vi "wsConnection_cycle_index.vi"() -> ()   [LabVIEW 2013]
uses:
  <vilib>/MediaMongrels Ltd/WebSockets/WebSockets/WebSockets.lvlib
panel:
  out "Numeric":i32
  in  "Frequency":dbl min=0.0
  in  "stop":bool
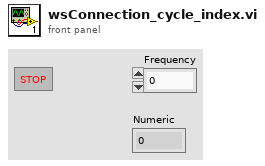
[diagram p1: front panel]
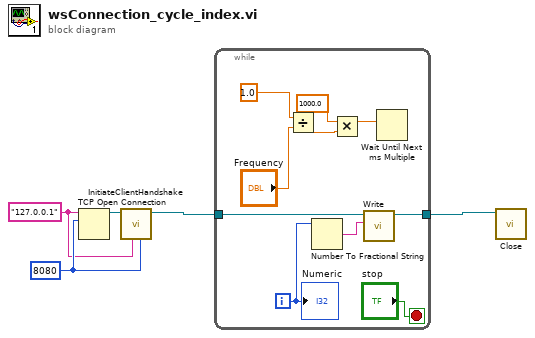
[diagram p0: block diagram]
diagram:
  w4 = "127.0.0.1"
  w5 = 8080
  n1 = TCP Open Connection(address=w4, remote port or service name=w5) -> (connection ID=w3:refnum<k5>)  [unwired: 3 in, 1 out]
  n2 = call <vilib>:"InitiateClientHandshake.vi"("remote port or service name"=w5, "address"=w4, "WebSocket Connection in"=w3) -> ("WebSocket Connection out"=w2:refnum<k5>)  [unwired: 6 in, 2 out]
  n3 = while {
    tunnel: [w13] -> w1
    tunnel: w2 -> [w12]
    i -> [w11]
    stop <- "stop" stop-if-true
    n4 = Divide(x=1.0, y="Frequency") -> (x/y=w7:dbl)
    n5 = Number To Fractional String(number=w11) -> (F-format string=w14:string)  [unwired: 3 in]
    n6 = Multiply(x=1000.0, y=w7) -> (x*y=w8:dbl)
    n7 = call <vilib>:"Write.vi"("Data"=w14, "WebSocket Connection in"=w12) -> ("WebSocket Connection out"=w13:refnum<k5>)  [unwired: 8 in, 1 out]
    n8 = Wait Until Next ms Multiple(millisecond multiple=w8) -> ()  [unwired: 1 out]
    "Numeric" <- w11
  }
  n9 = call <vilib>:"Close.vi"("WebSocket Connection in"=w1) -> ()  [unwired: 9 in, 2 out]
